vi "F23.vi"(8 "error in (no error)":errorcluster, 9 "data":u8[](array[numeric]), 10 "function":u8, 11 "device data model in":refnum<class "Standard Data Model.lvclass">) -> (0 "error out":errorcluster, 1 "data return":u8[](array[numeric]), 2 "function return":u8, 3 "device data model out":refnum<class "Standard Data Model.lvclass">)   [LabVIEW 2020, in "SubVIs.lvlib" / "Standard Data Model.lvclass"]
doc: "Executes function code 23"
uses:
  <vilib>/Modbus/subvis/Data and Functions/Standard Data Model/Standard Data Model.lvclass
  <vilib>/Modbus/subvis/SubVIs.lvlib
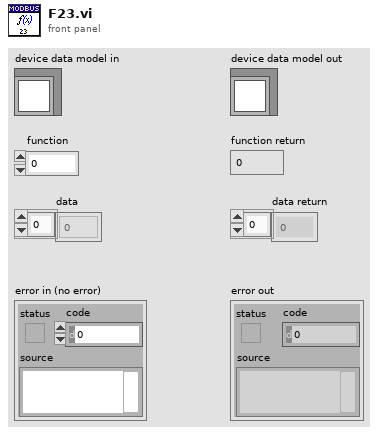
[diagram p1: front panel]
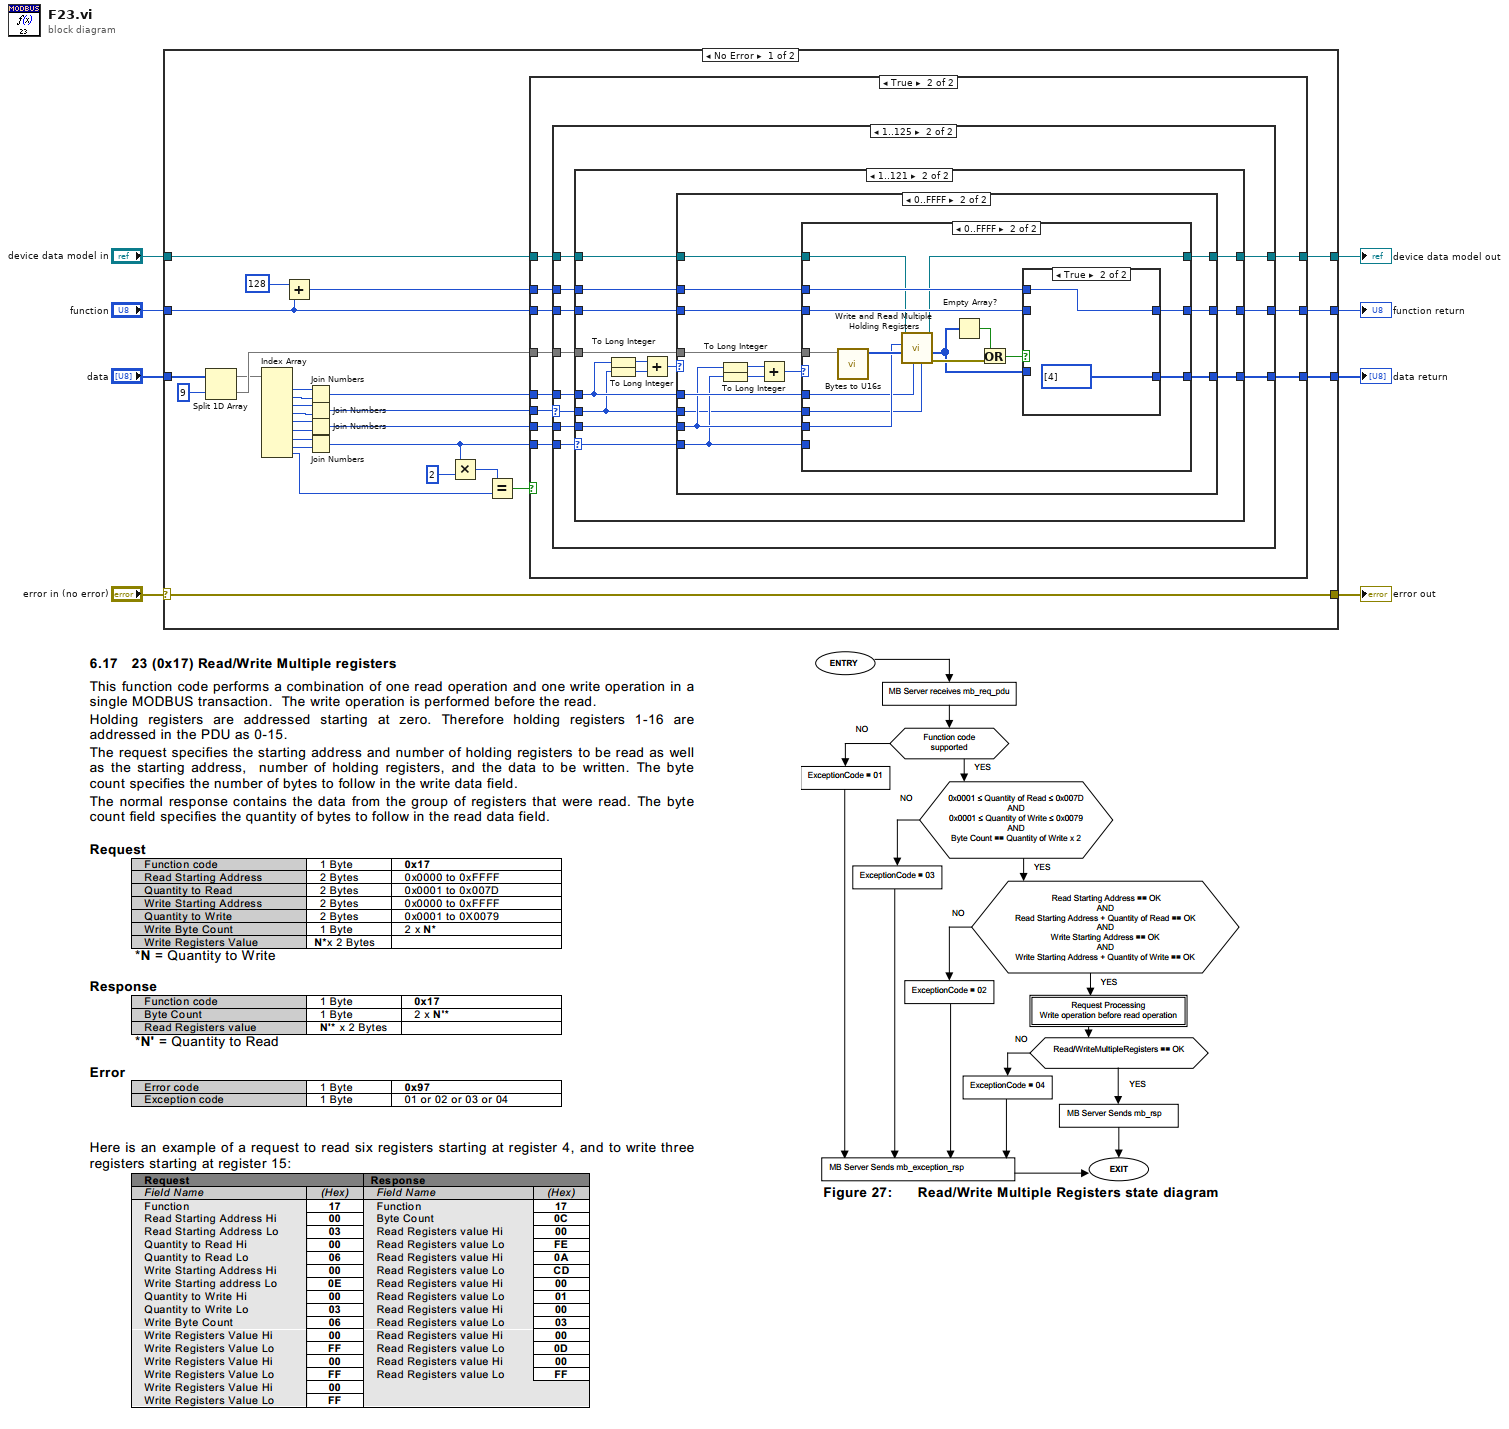
[diagram p0: block diagram]
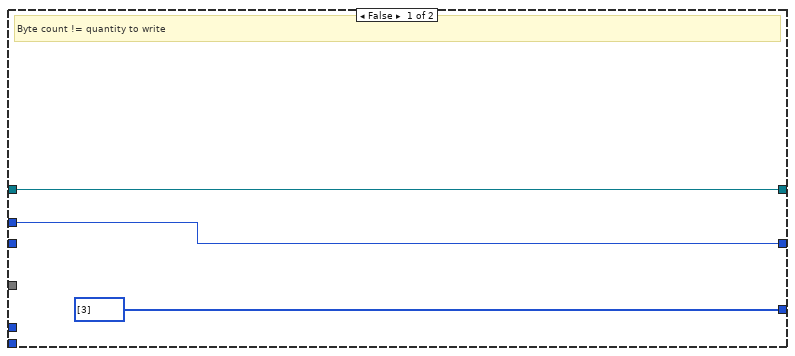
[diagram p2: hidden frame]
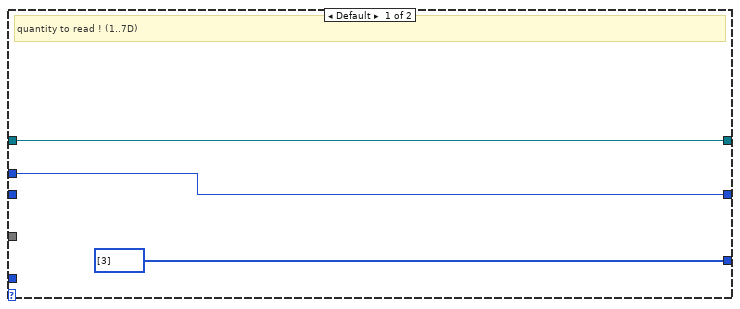
[diagram p3: hidden frame]
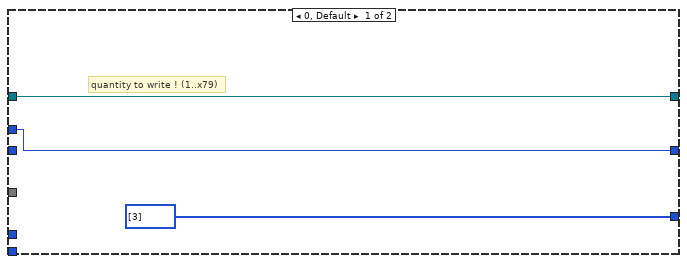
[diagram p4: hidden frame]
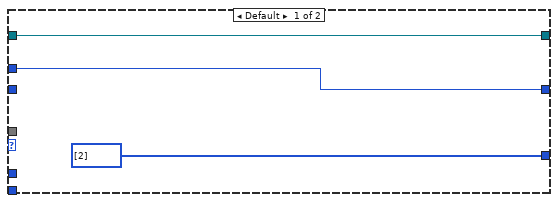
[diagram p5: hidden frame]
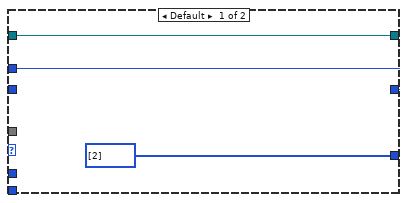
[diagram p6: hidden frame]
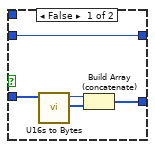
[diagram p7: hidden frame]
diagram:
  n1 = case shown="No Error" "error in (no error)" {
    selector: "error in (no error)" -> [w36 w127]
    tunnel: [w36 w127] -> w7
    tunnel: [w31 w126] -> w5
    tunnel: "device data model in" -> [w30 w126]
    tunnel: "function" -> [w27 w125]
    tunnel: "data" -> [w21 w124]
    tunnel: [w26 w125] -> w2
    tunnel: [w25 w124] -> w1
    frame No Error {
      n2 = Split 1D Array(array=w21, index=9) -> (first subarray=w18:u8[], second subarray=w19:u8[])
      n3 = Index Array(array=w18) -> (element #1=w34:u8, element #2=w35:u8, element #3=w33:u8, element #4=w32:u8, element #5=w14:u8, element #6=w13:u8, element #7=w11:u8, element #8=w12:u8, element #9=w15:u8)  [unwired: 9 in]
      n4 = Add(x=u8 128, y=w27) -> (x+y=w28:u8)
      n5 = Join Numbers(hi=w34, lo=w35) -> ((hi.lo)=w24:u16)
      n6 = Join Numbers(hi=w33, lo=w32) -> ((hi.lo)=w23:u16)
      n7 = Join Numbers(hi=w14, lo=w13) -> ((hi.lo)=w10:u16)
      n8 = Join Numbers(hi=w11, lo=w12) -> ((hi.lo)=w9:u16)
      n9 = Multiply(x=w9, y=u16 2) -> (x*y=w16:u16)
      n10 = Equal?(x=w16, y=w15) -> (x = y?=w17:bool)
      n11 = case shown="True" w17 {
        tunnel: w23 -> [_ w50]
        tunnel: [w39 w49] -> w31
        tunnel: w30 -> [w39 w48]
        tunnel: w28 -> [w38 w47]
        tunnel: w27 -> [_ w46]
        tunnel: [w38 w45] -> w26
        tunnel: [u8[] [3] ("Data Return") w44] -> w25
        tunnel: w24 -> [_ w43]
        tunnel: w19 -> [_ w42]
        tunnel: w10 -> [_ w40]
        tunnel: w9 -> [_ w41]
        frame False {
          # "Byte count != quantity to write"
        }
        frame True {
          n12 = case shown="1..125" w50 {
            selector: w50 -> [_ w63]
            tunnel: [w53 w62] -> w49
            tunnel: w48 -> [w53 w61]
            tunnel: w47 -> [w52 w60]
            tunnel: w46 -> [_ w58]
            tunnel: [w52 w59] -> w45
            tunnel: [u8[] [3] ("Data Return") w57] -> w44
            tunnel: w43 -> [_ w64]
            tunnel: w42 -> [_ w56]
            tunnel: w41 -> [_ w55]
            tunnel: w40 -> [_ w54]
            frame Default {
              # "quantity to read ! (1..7D)"
            }
            frame 1..125 {
              n13 = case shown="1..121" w55 {
                selector: w55 -> [_ w68]
                tunnel: w64 -> [_ w78]
                tunnel: w63 -> [_ w77]
                tunnel: [w66 w76] -> w62
                tunnel: w61 -> [w66 w75]
                tunnel: w60 -> [w65 w74]
                tunnel: [w65 w73] -> w59
                tunnel: w58 -> [_ w72]
                tunnel: [u8[] [3] ("Data Return") w71] -> w57
                tunnel: w56 -> [_ w70]
                tunnel: w54 -> [_ w69]
                frame 0, Default {
                  # "quantity to write ! (1..x79)"
                }
                frame 1..121 {
                  n14 = To Long Integer(number=w78) -> (32bit integer=w81:i32)
                  n15 = To Long Integer(number=w77) -> (32bit integer=w80:i32)
                  n16 = Add(x=w81, y=w80) -> (x+y=w79:i32)
                  n17 = case shown="0..FFFF" w79 {
                    tunnel: w78 -> [_ w92]
                    tunnel: w77 -> [_ w85]
                    tunnel: [w84 w98] -> w76
                    tunnel: w75 -> [w84 w93]
                    tunnel: w74 -> [w83 w97]
                    tunnel: [w83 w95] -> w73
                    tunnel: w72 -> [_ w96]
                    tunnel: [u8[] [2] ("Data Return") w94] -> w71
                    tunnel: w70 -> [_ w91]
                    tunnel: w69 -> [_ w87]
                    tunnel: w68 -> [_ w86]
                    frame Default {
                    }
                    frame 0..65535 {
                      n18 = To Long Integer(number=w87) -> (32bit integer=w89:i32)
                      n19 = To Long Integer(number=w86) -> (32bit integer=w90:i32)
                      n20 = Add(x=w89, y=w90) -> (x+y=w88:i32)
                      n21 = case shown="0..FFFF" w88 {
                        tunnel: [w100 w102] -> w98
                        tunnel: w97 -> [w99 w116]
                        tunnel: w96 -> [_ w115]
                        tunnel: [w99 w114] -> w95
                        tunnel: [u8[] [2] ("Data Return") w113] -> w94
                        tunnel: w93 -> [w100 w110]
                        tunnel: w92 -> [_ w103]
                        tunnel: w91 -> [_ w112]
                        tunnel: w87 -> [_ w108]
                        tunnel: w86 -> [_ _]
                        tunnel: w85 -> [_ w107]
                        frame Default {
                        }
                        frame 0..65535 {
                          n22 = call <vilib>:"Bytes to U16s.vi"("bytes"=w112) -> ("registers"=w109:u16[])  [unwired: 10 in]
                          n23 = call-dynamic "Write and Read Multiple Holding Registers.vi"("read count"=w107, "read starting address"=w103, "write values"=w109, "write starting address"=w108, "device data model in"=w110) -> ("error out"=w111:errorcluster, "read values"=w104:u16[], "device data model out"=w102:refnum<class "Standard Data Model.lvclass">)  [unwired: 4 in]
                          n24 = Empty Array?(array=w104) -> (empty?=w105:bool)
                          n25 = Or(x=w105, y=w111) -> (x .or. y?=w106:bool)
                          n26 = case shown="True" w106 {
                            tunnel: w116 -> [_ w123]
                            tunnel: w115 -> [w121 _]
                            tunnel: [w121 w123] -> w114
                            tunnel: [w117 u8[] [4]] -> w113
                            tunnel: w104 -> [w120 _]
                            frame False {
                              n27 = call <vilib>:"U16s to Bytes.vi"("registers"=w120) -> ("bytes"=w118:u8[], "count"=w119:u8)  [unwired: 9 in]
                              n28 = Build Array (concatenate)(w119, w118) -> (w117:u8[])
                            }
                            frame True {
                            }
                          }
                        }
                      }
                    }
                  }
                }
              }
            }
          }
        }
      }
    }
    frame Error {
    }
  }
  "error out" <- w7
  "device data model out" <- w5
  "data return" <- w1
  "function return" <- w2
